vi "Strafe.vi"(8 "X target":dbl, 10 "Encoders In":T1, 11 "PID Gains In":T2={"X PID"={"proportional gain (Kc)"=0.02000000000000001, "integral time (Ti, min)"=0.0, "derivative time (Td, min)"=0.0}, "Y PID"={"proportional gain (Kc)"=0.02000000000000001, "integral time (Ti, min)"=0.0, "derivative time (Td, min)"=0.0}, "Z PID"={"proportional gain (Kc)"=0.02000000000000001, "integral time (Ti, min)"=0.0, "derivative time (Td, min)"=0.0}} {"Z PID"."derivative time (Td, min)" format="%.3f"; "Z PID"."integral time (Ti, min)" format="%.3f"; "Z PID"."proportional gain (Kc)" format="%.3f"; "Y PID"."derivative time (Td, min)" format="%.3f"; "Y PID"."integral time (Ti, min)" format="%.3f"; "Y PID"."proportional gain (Kc)" format="%.3f"; "X PID"."derivative time (Td, min)" format="%.3f"; "X PID"."integral time (Ti, min)" format="%.3f"; "X PID"."proportional gain (Kc)" format="%.3f"}) -> (2 "Encoders Out":T1, 3 "PID Gains Out":T2={"X PID"={"proportional gain (Kc)"=0.02000000000000001, "integral time (Ti, min)"=0.0, "derivative time (Td, min)"=0.0}, "Y PID"={"proportional gain (Kc)"=0.02000000000000001, "integral time (Ti, min)"=0.0, "derivative time (Td, min)"=0.0}, "Z PID"={"proportional gain (Kc)"=0.02000000000000001, "integral time (Ti, min)"=0.0, "derivative time (Td, min)"=0.0}} {"Z PID"."derivative time (Td, min)" format="%.3f"; "Z PID"."integral time (Ti, min)" format="%.3f"; "Z PID"."proportional gain (Kc)" format="%.3f"; "Y PID"."derivative time (Td, min)" format="%.3f"; "Y PID"."integral time (Ti, min)" format="%.3f"; "Y PID"."proportional gain (Kc)" format="%.3f"; "X PID"."derivative time (Td, min)" format="%.3f"; "X PID"."integral time (Ti, min)" format="%.3f"; "X PID"."proportional gain (Kc)" format="%.3f"})   [LabVIEW 2018]
uses:
  <vilib>/addons/control/pid/NI_PID_pid.lvlib
  Robot Global Data.vi
  <vilib>/addons/control/pid/pid.llb/PID (DBL).vi
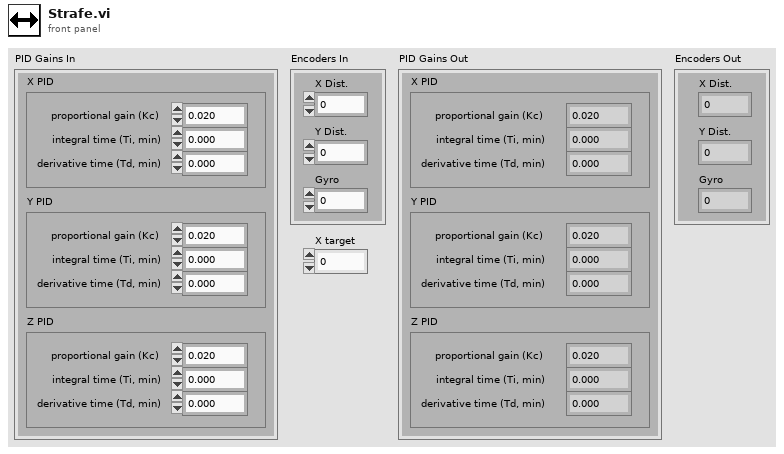
[diagram p1: front panel]
types:
  T1 = cluster{"X Dist.":dbl, "Y Dist.":dbl, "Gyro":dbl}
  T2 = cluster{"X PID":cluster{"proportional gain (Kc)":dbl, "integral time (Ti, min)":dbl, "derivative time (Td, min)":dbl}, "Y PID":cluster{"proportional gain (Kc)":dbl, "integral time (Ti, min)":dbl, "derivative time (Td, min)":dbl}, "Z PID":cluster{"proportional gain (Kc)":dbl, "integral time (Ti, min)":dbl, "derivative time (Td, min)":dbl}}
  T3 = cluster{"proportional gain (Kc)":dbl, "integral time (Ti, min)":dbl, "derivative time (Td, min)":dbl}
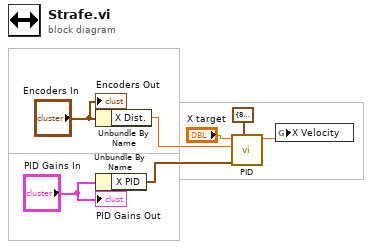
[diagram p0: block diagram]
diagram:
  n1 = Unbundle By Name("Encoders In") -> ("X Dist."=w2:dbl)
  n2 = Unbundle By Name("PID Gains In") -> ("X PID"=w1:T3)
  n3 = call-poly <vilib>:"PID.vi"("output range"=cluster{"output high":dbl, "output low":dbl} {"output high"=8.0, "output low"=-8.0}, "PID gains"=w1, "process variable"=w2, "setpoint"="X target") -> ("output"=w5:dbl)  [unwired: 6 in, 1 out]
  n4 = global write "Robot Global Data.vi" "X Velocity"(w5) -> ()
  "PID Gains Out" <- "PID Gains In"
  "Encoders Out" <- "Encoders In"
